vi "APLUS Camille Bauer Driver.vi"(8 "error in (no error)":errorcluster, 9 "Reset WattHours":bool, 10 "Remote Port":u16=502, 11 "Remote IP Address":string="192.168.1.101") -> (0 "error out":errorcluster, 3 "output cluster":T1)   [LabVIEW 2012]
uses:
  <vilib>/NI Modbus.llb/MB Ethernet Master Query Read Holding Registers (poly).vi
  <vilib>/NI Modbus.llb/MB Ethernet Master Query Write Single Coil (poly).vi
panel:
  in  "Watt Hour Reset Register":u16=1459
  out "Holding Registers":u16[](array[numeric])
  # "TCP Parameters"
  # "Data to write to the slave"
  # "Slave Read-only Registers"
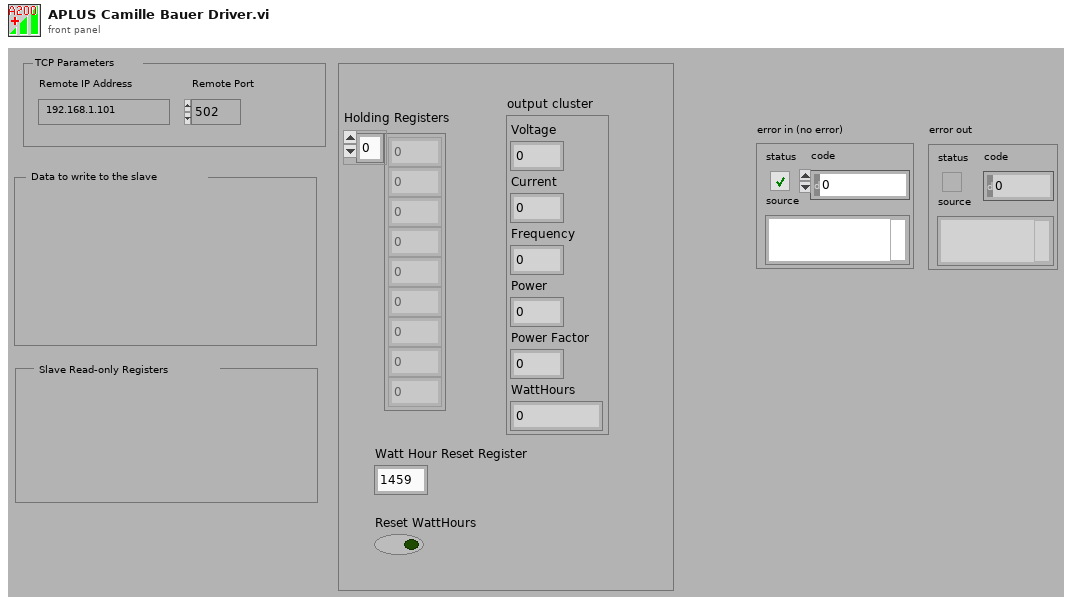
[diagram p1: front panel]
types:
  T1 = cluster{"Voltage":sgl, "Current":sgl, "Frequency":sgl, "Power":sgl, "Power Factor":sgl, "WattHours":sgl}
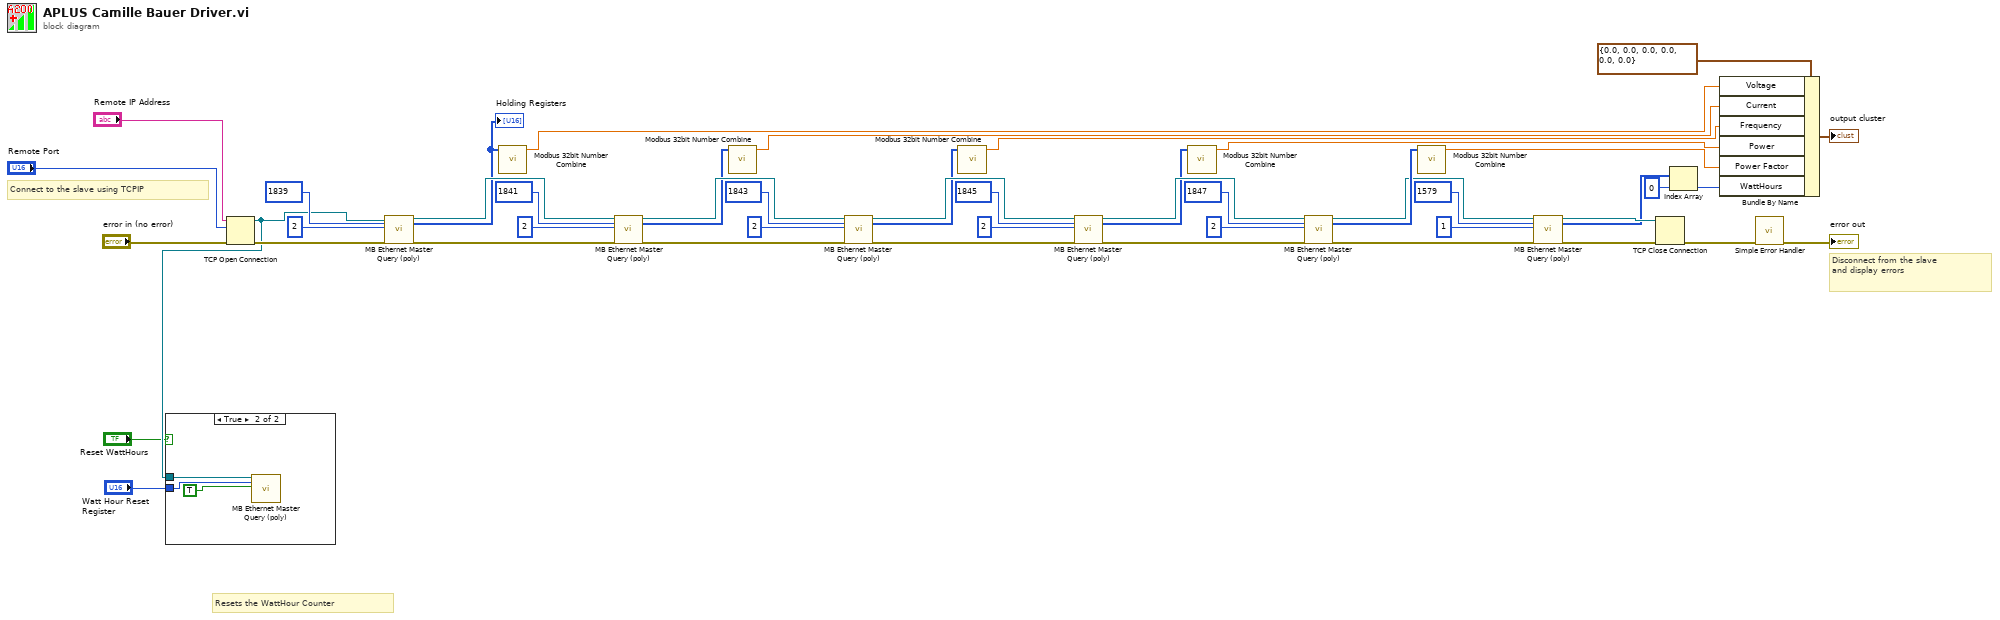
[diagram p0: block diagram]
diagram:
  # "Resets the WattHour Counter"
  # "Disconnect from the slave\nand display errors"
  # "Connect to the slave using TCPIP"
  n1 = TCP Open Connection(address="Remote IP Address", remote port or service name="Remote Port", error in (no error)="error in (no error)") -> (connection ID=w2:refnum<k5>, error out=w14:errorcluster)  [unwired: 2 out]
  n2 = case shown="True" "Reset WattHours" {
    tunnel: "Watt Hour Reset Register" -> [_ w50]
    tunnel: w2 -> [_ w51]
    frame False {
    }
    frame True {
      n3 = call-poly <vilib>:"MB Ethernet Master Query (poly).vi"("TCP Connection Refnum in"=w51, "Address"=w50, "Coil"=TRUE) -> ()  [unwired: 3 in, 14 out]
    }
  }
  n4 = call-poly <vilib>:"MB Ethernet Master Query (poly).vi"("TCP Connection Refnum in"=w2, "Starting Address"=u16 1839, "Quantity"=u16 2, "error in"=w14) -> ("TCP Connection Refnum (dup)"=w30:refnum<k5>, "Holding Registers"=w17:u16[], "error out"=w20:errorcluster)  [unwired: 1 in, 12 out]
  "Holding Registers" <- w17
  n5 = call "Modbus 32bit Number Combine.vi"("Holding Registers"=w17) -> ("Numeric"=w39:sgl)  [unwired: 10 in]
  n6 = call-poly <vilib>:"MB Ethernet Master Query (poly).vi"("TCP Connection Refnum in"=w30, "Starting Address"=u16 1841, "Quantity"=u16 2, "error in"=w20) -> ("TCP Connection Refnum (dup)"=w31:refnum<k5>, "Holding Registers"=w27:u16[], "error out"=w18:errorcluster)  [unwired: 1 in, 12 out]
  n7 = call "Modbus 32bit Number Combine.vi"("Holding Registers"=w27) -> ("Numeric"=w40:sgl)  [unwired: 10 in]
  n8 = call-poly <vilib>:"MB Ethernet Master Query (poly).vi"("TCP Connection Refnum in"=w31, "Starting Address"=u16 1843, "Quantity"=u16 2, "error in"=w18) -> ("TCP Connection Refnum (dup)"=w32:refnum<k5>, "Holding Registers"=w28:u16[], "error out"=w19:errorcluster)  [unwired: 1 in, 12 out]
  n9 = call "Modbus 32bit Number Combine.vi"("Holding Registers"=w28) -> ("Numeric"=w41:sgl)  [unwired: 10 in]
  n10 = call-poly <vilib>:"MB Ethernet Master Query (poly).vi"("TCP Connection Refnum in"=w32, "Starting Address"=u16 1845, "Quantity"=u16 2, "error in"=w19) -> ("TCP Connection Refnum (dup)"=w37:refnum<k5>, "Holding Registers"=w29:u16[], "error out"=w33:errorcluster)  [unwired: 1 in, 12 out]
  n11 = call "Modbus 32bit Number Combine.vi"("Holding Registers"=w29) -> ("Numeric"=w42:sgl)  [unwired: 10 in]
  n12 = call-poly <vilib>:"MB Ethernet Master Query (poly).vi"("TCP Connection Refnum in"=w37, "Starting Address"=u16 1847, "Quantity"=u16 2, "error in"=w33) -> ("TCP Connection Refnum (dup)"=w9:refnum<k5>, "Holding Registers"=w36:u16[], "error out"=w13:errorcluster)  [unwired: 1 in, 12 out]
  n13 = call "Modbus 32bit Number Combine.vi"("Holding Registers"=w36) -> ("Numeric"=w43:sgl)  [unwired: 10 in]
  n14 = call-poly <vilib>:"MB Ethernet Master Query (poly).vi"("TCP Connection Refnum in"=w9, "Starting Address"=u16 1579, "Quantity"=u16 1, "error in"=w13) -> ("TCP Connection Refnum (dup)"=w8:refnum<k5>, "Holding Registers"=w6:u16[], "error out"=w12:errorcluster)  [unwired: 1 in, 12 out]
  n15 = TCP Close Connection(connection ID=w8, error in (no error)=w12) -> (error out=w46:errorcluster)  [unwired: 2 out]
  n16 = Index Array(array=w6, index=0) -> (element=w4:u16)
  n17 = Bundle By Name(cluster=T1 {"Voltage"=0.0, "Current"=0.0, "Frequency"=0.0, "Power"=0.0, "Power Factor"=0.0, "WattHours"=0.0} ("input cluster"), "Voltage"=w39, "Current"=w40, "Frequency"=w41, "Power"=w42, "Power Factor"=w43, "WattHours"=w4) -> (→"output cluster":T1)
  n18 = call <vilib>:"Simple Error Handler.vi"("error in (no error)"=w46) -> ("error out"=→"error out":errorcluster)  [unwired: 1 in, 7 out]
